vi "Public SV.vi"(0 "reference in":refnum<class "Stand.lvclass">, 11 "error in (no error)":errorcluster) -> (4 "reference out":refnum<class "Stand.lvclass">, 12 "dt public sv":u32, 15 "error out":errorcluster)   [LabVIEW 2019, in "Stand.lvclass"]
uses:
  Stand.lvclass
  C:/Users/ANENKOV_V1/Desktop/src/Device_class/Device.lvclass
  Stand.lvclass/Stand.ctl
  Device_class/Device.lvclass/Device.ctl
  DI_class/DI.lvclass/DI.ctl
  SV_Puplisher_class/SV_Publisher.lvclass/SV_Publisher.ctl
  FPGA/TypeDef/AI index.ctl
  AI_class/AI.lvclass/AI.ctl
  AnalogComparator_class/AnalogComparator.lvclass/AnalogComparator.ctl
  TypeDef/State Engine.ctl
  PM_Group_class/PM_Group.lvclass/PM_Group.ctl
  Engine_1DO_2DI_class/Engine_1DO_2DI.lvclass/Engine_1DO_2DI.ctl
  Valve_2DO_2DI_class/Valve_2DO_2DI.lvclass/Valve_2DO_2DI.ctl
  SV_Puplisher_class/Set SV.vi/1ae5d02c-efd0-450a-8aa4-8388e25d05bc.vi
  AnalogComparator_class/GetStatus.vi
  Engine_1DO_2DI_class/GetEngineState.vi
  Engine_1DO_2DI_class/Engine_1DO_2DI.lvclass
  OWEN HMI/Global - Data.vi
  FPGA_API_class/FPGA API.lvclass
  AI_class/AI.lvclass
  DI_class/DI.lvclass
  SV_Puplisher_class/SV_Publisher.lvclass
  Device_class/Device.lvclass
  PM_Group_class/PM_Group.lvclass
  ExpFitter/ExpFitter.lvclass
  OWEN HMI/OWEN HMI.lvclass
  Valve_2DO_2DI_class/Valve_2DO_2DI.lvclass
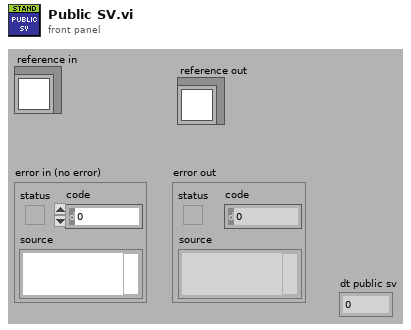
[diagram p1: front panel]
types:
  T1 = typedef "AI index.ctl" = u8
  T2 = typedef "AI_Data.ctl" = cluster{"Stat Data":T3, "OutOfRangeMax":bool, "OutOfRangeMin":bool, "HIHI":bool, "HI":bool, "LO":bool, "LOLO":bool}
  T3 = typedef "AI Statistics Data.ctl" = cluster{"raw mean":dbl, "scl mean":dbl, "raw mean 1Hz":dbl, "scl mean 1Hz":dbl}
  T4 = typedef "State Engine.ctl" = enum16{"Unknown", "Off", "TupningOn", "On", "TurningOff"}
  T5 = typedef "State PMG.ctl" = cluster{"PMG Mode":T6, "M12":T7, "M21":T7, "M24":T7}
  T6 = typedef "PMG Mode.ctl" = enum16{"Idel", "Filling", "Pressure"}
  T7 = typedef "State Engine 2.ctl" = cluster{"EngState":T4, "Active":bool, "Contactor":bool, "CMD":bool, "Automat":bool}
  T8 = typedef "Data Stand.ctl" = cluster{"CommCounter":u64, "BeginFilingLevel":dbl, "SP DUT":dbl, "SP CHAMBER":dbl, "Mode":T9, "ExecuteStepState":T10, "Direction":T11, "Direction Filling":T11, "STS":T12, "SP_TYPE_DUT":T13, "SP_TYPE_CHAMBER":T13, "New Step":bool, "BURETE_TIME":u16, "With BURETE":bool, "With Nitro":bool, "State 44-1-2":T14, "Measure leak":bool, "hold":bool}
  T9 = typedef "Mode.ctl" = enum16{"IDLE", "FILLING", "EXECUTE_SP", "DRAIN"}
  T10 = typedef "ExecuteStepState.ctl" = enum16{"Init", "Set: Backpressure ", "Preload: HI", "Set: HI", "Maintenance: HI", "Down: Pressure", "BLOCK"}
  T11 = typedef "Direction.ctl" = enum8{"DUT", "Chamber"}
  T12 = typedef "STS REG.ctl" = cluster{"IDLE":bool, "RYADY":bool, "STEP":bool, "ALARM":bool, "WARNING":bool, "REMOTE":bool, "SP_EXEC_DONE_DUT":bool, "SP_EXEC_DONE_CHAMBER":bool, "FILING_DONE_DUT":bool, "FILING_DONE_CHAMBER":bool, "BURETE_STATE":bool}
  T13 = typedef "SP_TYPE.ctl" = enum16{"ERROR", "ZIRO", "BASE", "SP"}
  T14 = typedef "State 44-1-2.ctl" = enum16{"Init", "Idle", "Wait", "Open 44-1", "Open 44-2", "Close 44-1", "Close 44-2"}
  T15 = typedef "DataExpFit.ctl" = cluster{"amplitude":dbl, "damping":dbl, "offset":dbl, "residue":dbl, "valid":bool, "T [s]":dbl}
  T16 = typedef "valveState.ctl" = enum16{"Unknown", "Closed", "Opening", "Opened", "Closing"}
  T17 = typedef "Setting Stand.ctl" = cluster{"Pressure Source":T18, "dt pressure down ms":i32, "dP pressure down MPa":dbl, "Haskel":T19, "Pump":T19, "Accuracy [%]":dbl, "Accuracy max [MPa]":dbl, "Accuracy min [MPa]":dbl, "BackPressurVoltage [V]":dbl}
  T18 = typedef "Pressure Source.ctl" = enum16{"Internal", "Modbus", "UDP"}
  T19 = typedef "Setting Pressure PI.ctl" = cluster{"A [MPa/V]":dbl, "P0 [MPa]":dbl}
  T20 = typedef "TCP Slave.lvclass/Connection.ctl" = cluster{"Connected?":bool, "IP address":string, "connection error":errorcluster}
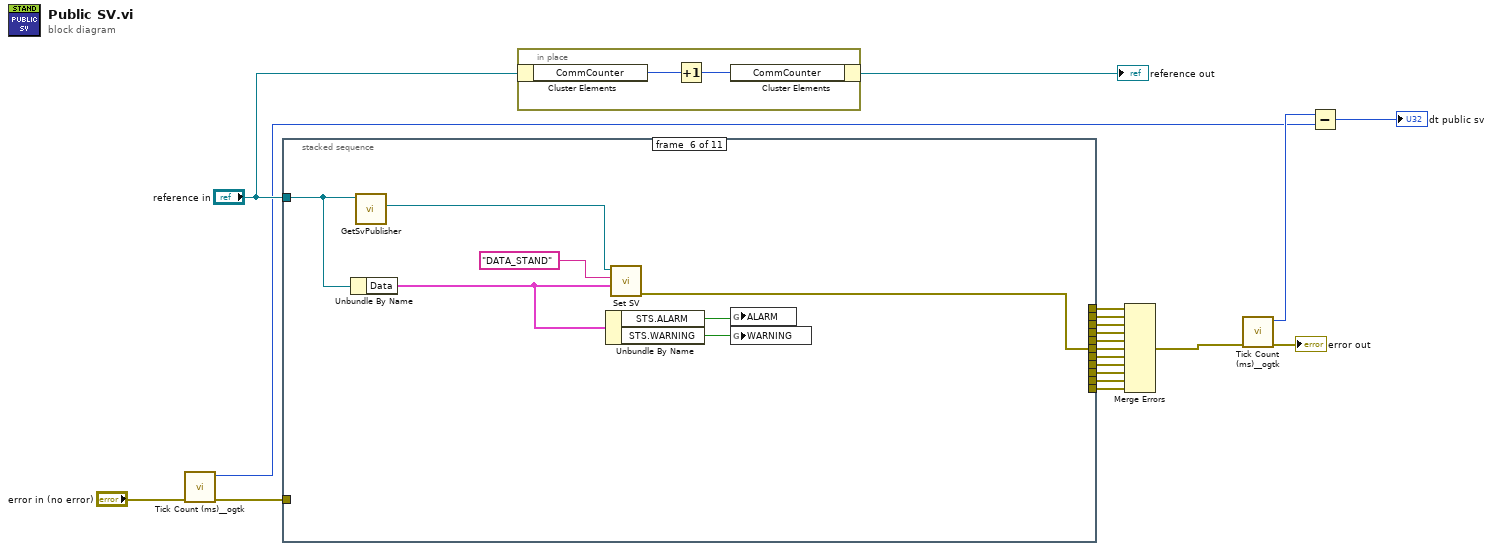
[diagram p0: block diagram]
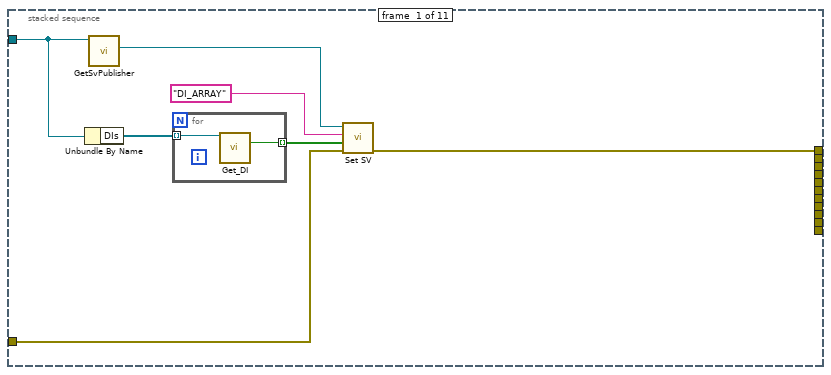
[diagram p2: hidden frame]
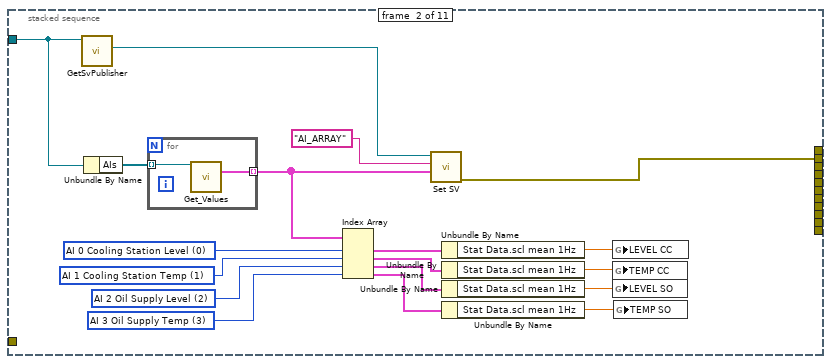
[diagram p3: hidden frame]
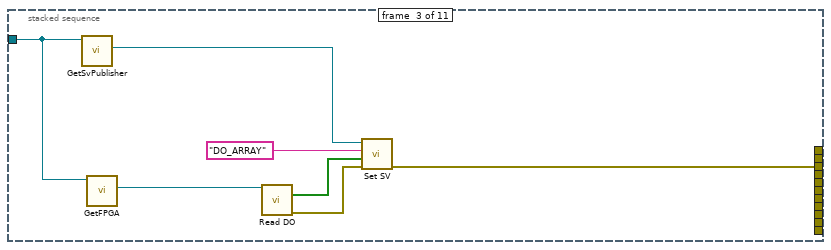
[diagram p4: hidden frame]
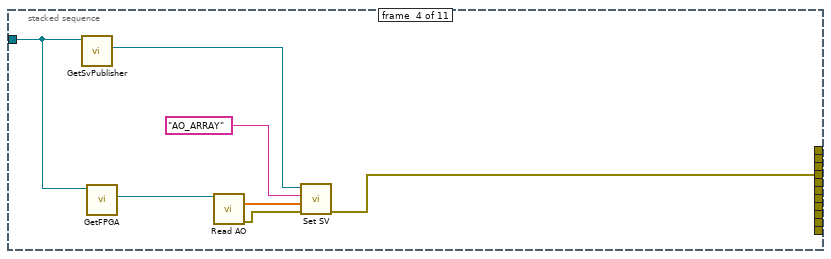
[diagram p5: hidden frame]
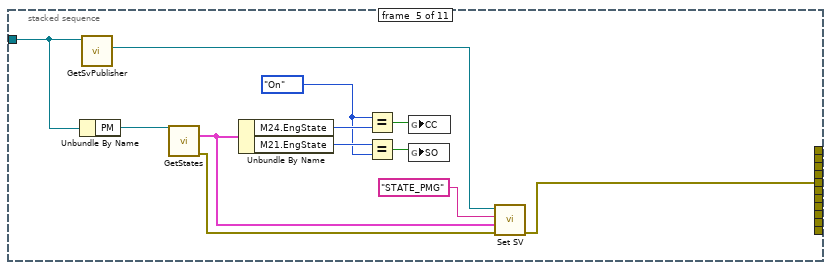
[diagram p6: hidden frame]
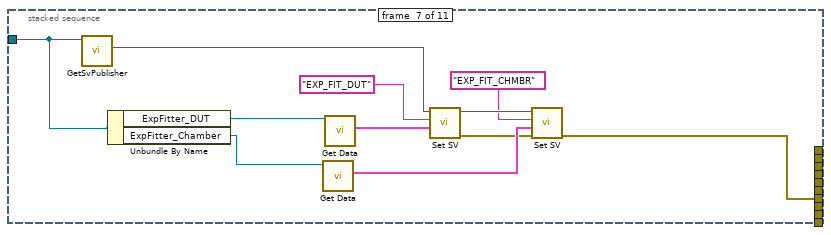
[diagram p7: hidden frame]
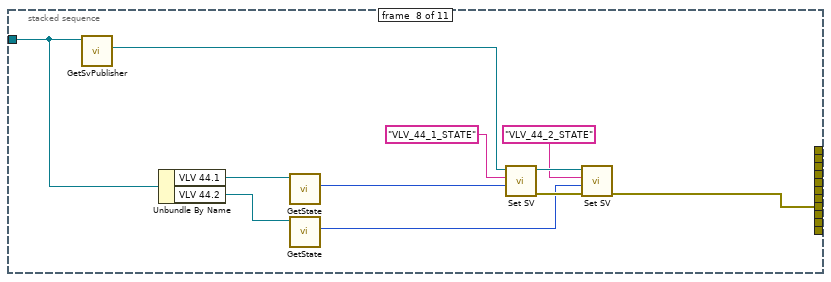
[diagram p8: hidden frame]
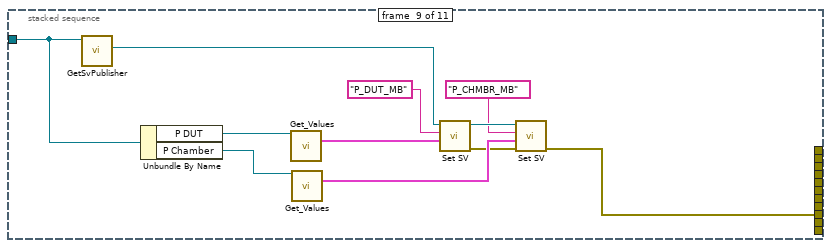
[diagram p9: hidden frame]
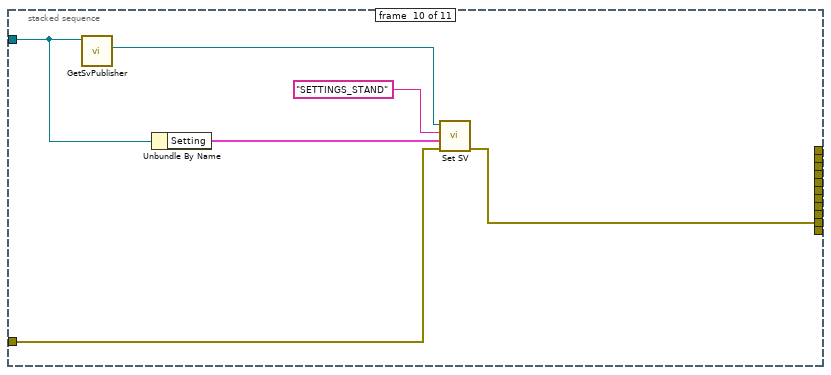
[diagram p10: hidden frame]
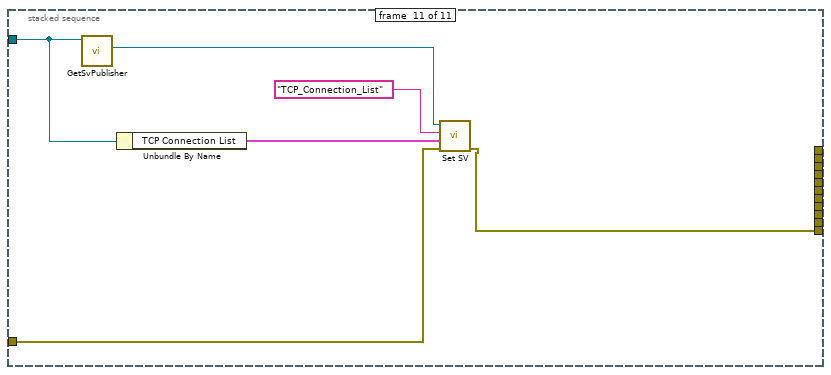
[diagram p11: hidden frame]
diagram:
  n1 = call <userlib>:"Tick Count (ms)__ogtk.vi"("error in (no error)"="error in (no error)") -> ("error out"=w13:errorcluster, "millisecond timer value"=w14:u32)  [unwired: 9 in]
  n2 = stacked-sequence {
    tunnel: "reference in" -> [w25 w47 w54 w63 w75 w82 w93 w96 w107 w120 w126]
    tunnel: w13 -> [w21 _ _ _ _ _ _ _ _ w116 w123]
    tunnel: [w22 _ _ _ _ _ _ _ _ _ _] -> w12
    tunnel: [_ w30 _ _ _ _ _ _ _ _ _] -> w10
    tunnel: [_ _ w50 _ _ _ _ _ _ _ _] -> w9
    tunnel: [_ _ _ w57 _ _ _ _ _ _ _] -> w8
    tunnel: [_ _ _ _ w64 _ _ _ _ _ _] -> w7
    tunnel: [_ _ _ _ _ w79 _ _ _ _ _] -> w6
    tunnel: [_ _ _ _ _ _ w83 _ _ _ _] -> w5
    tunnel: [_ _ _ _ _ _ _ w94 _ _ _] -> w4
    tunnel: [_ _ _ _ _ _ _ _ w105 _ _] -> w3
    tunnel: [_ _ _ _ _ _ _ _ _ w117 _] -> w2
    tunnel: [_ _ _ _ _ _ _ _ _ _ w122] -> w1
    frame #0 {
      n3 = Unbundle By Name(w25) -> ("DIs"=w24:refnum<class "DI.lvclass">[])
      n4 = call "GetSvPublisher.vi"("Device in"=w25) -> ("SV_Publisher.lvclass"=w23:refnum<class "SV_Publisher.lvclass">)  [unwired: 10 in]
      n5 = for {
        tunnel: w24 -> [w29] mode=indexing
        tunnel: [w28] -> w27 mode=indexing
        n6 = call "Get_DI.vi"("reference in"=w29) -> ("DI"=w28:bool)  [unwired: 14 in]
      }
      n7 = call "Set SV.vi"("error in (no error)"=w21, "SV Value"=w27, "SV Name"="DI_ARRAY", "SV_Publisher in"=w23) -> ("error out"=w22:errorcluster)  [unwired: 6 in, 1 out]
    }
    frame #1 {
      w34 = T1 3 items=["AI 0 Cooling Station Level", "AI 1 Cooling Station Temp", "AI 2 Oil Supply Level", "AI 3 Oil Supply Temp", "AI 4 ", "AI 5 Pressure Haskel", "AI 6 Pressure DUT", "AI 7 Pressure Chamber", "AI 8 Pressure Air inlet", "AI 9 Pressure Air outlet", "AI 10 Pressure Messure Line"] ("AI index")
      w35 = T1 2 items=["AI 0 Cooling Station Level", "AI 1 Cooling Station Temp", "AI 2 Oil Supply Level", "AI 3 Oil Supply Temp", "AI 4 ", "AI 5 Pressure Haskel", "AI 6 Pressure DUT", "AI 7 Pressure Chamber", "AI 8 Pressure Air inlet", "AI 9 Pressure Air outlet", "AI 10 Pressure Messure Line"] ("AI index")
      w36 = T1 1 items=["AI 0 Cooling Station Level", "AI 1 Cooling Station Temp", "AI 2 Oil Supply Level", "AI 3 Oil Supply Temp", "AI 4 ", "AI 5 Pressure Haskel", "AI 6 Pressure DUT", "AI 7 Pressure Chamber", "AI 8 Pressure Air inlet", "AI 9 Pressure Air outlet", "AI 10 Pressure Messure Line"] ("AI index")
      w37 = T1 0 items=["AI 0 Cooling Station Level", "AI 1 Cooling Station Temp", "AI 2 Oil Supply Level", "AI 3 Oil Supply Temp", "AI 4 ", "AI 5 Pressure Haskel", "AI 6 Pressure DUT", "AI 7 Pressure Chamber", "AI 8 Pressure Air inlet", "AI 9 Pressure Air outlet", "AI 10 Pressure Messure Line"] ("AI index")
      n8 = call "GetSvPublisher.vi"("Device in"=w47) -> ("SV_Publisher.lvclass"=w31:refnum<class "SV_Publisher.lvclass">)  [unwired: 10 in]
      n9 = Unbundle By Name(w47) -> ("AIs"=w32:refnum<class "AI.lvclass">[])
      n10 = for {
        tunnel: w32 -> [w49] mode=indexing
        tunnel: [w48] -> w38 mode=indexing
        n11 = call "Get_Values.vi"("reference in"=w49) -> ("Data"=w48:T2)  [unwired: 14 in]
      }
      n12 = Index Array(array=w38, index #1=w37, index #2=w36, index #3=w35, index #4=w34) -> (element #1=w39:T2, element #2=w40:T2, element #3=w41:T2, element #4=w42:T2)
      n13 = call "Set SV.vi"("SV Value"=w38, "SV Name"="AI_ARRAY", "SV_Publisher in"=w31) -> ("error out"=w30:errorcluster)  [unwired: 7 in, 1 out]
      n14 = Unbundle By Name(w39) -> ("Stat Data.scl mean 1Hz"=w43:dbl)
      n15 = Unbundle By Name(w40) -> ("Stat Data.scl mean 1Hz"=w46:dbl)
      n16 = Unbundle By Name(w41) -> ("Stat Data.scl mean 1Hz"=w45:dbl)
      n17 = Unbundle By Name(w42) -> ("Stat Data.scl mean 1Hz"=w44:dbl)
      n18 = global write "Global - Data.vi" "LEVEL CC"(w43) -> ()
      n19 = global write "Global - Data.vi" "TEMP CC"(w46) -> ()
      n20 = global write "Global - Data.vi" "LEVEL SO"(w45) -> ()
      n21 = global write "Global - Data.vi" "TEMP SO"(w44) -> ()
    }
    frame #2 {
      n22 = call "GetSvPublisher.vi"("Device in"=w54) -> ("SV_Publisher.lvclass"=w52:refnum<class "SV_Publisher.lvclass">)  [unwired: 10 in]
      n23 = call "GetFPGA.vi"("Device in"=w54) -> ("FPGA API.lvclass"=w53:refnum<class "FPGA API.lvclass">)  [unwired: 10 in]
      n24 = call-dynamic "Read DO.vi"("FPGA API in"=w53) -> ("Ds"=w56:bool[], "error out"=w51:errorcluster)  [unwired: 12 in, 1 out]
      n25 = call "Set SV.vi"("error in (no error)"=w51, "SV Value"=w56, "SV Name"="DO_ARRAY", "SV_Publisher in"=w52) -> ("error out"=w50:errorcluster)  [unwired: 6 in, 1 out]
    }
    frame #3 {
      n26 = call "GetSvPublisher.vi"("Device in"=w63) -> ("SV_Publisher.lvclass"=w59:refnum<class "SV_Publisher.lvclass">)  [unwired: 10 in]
      n27 = call "GetFPGA.vi"("Device in"=w63) -> ("FPGA API.lvclass"=w60:refnum<class "FPGA API.lvclass">)  [unwired: 10 in]
      n28 = call-dynamic "Read AO.vi"("FPGA API in"=w60) -> ("AO"=w62:dbl[], "error out"=w58:errorcluster)  [unwired: 12 in, 1 out]
      n29 = call "Set SV.vi"("error in (no error)"=w58, "SV Value"=w62, "SV Name"="AO_ARRAY", "SV_Publisher in"=w59) -> ("error out"=w57:errorcluster)  [unwired: 6 in, 1 out]
    }
    frame #4 {
      w69 = State_Engine."On" ("x")
      n30 = Unbundle By Name(w75) -> ("PM"=w67:refnum<class "PM_Group.lvclass">)
      n31 = call "GetSvPublisher.vi"("Device in"=w75) -> ("SV_Publisher.lvclass"=w65:refnum<class "SV_Publisher.lvclass">)  [unwired: 10 in]
      n32 = call "GetStates.vi"("Pump_1AI_1DO_2DI in"=w67) -> ("PMG"=w74:T5, "error out"=w66:errorcluster)  [unwired: 13 in]
      n33 = Unbundle By Name(w74) -> ("M24.EngState"=w70:T4, "M21.EngState"=w72:T4)
      n34 = Equal?(x=w69, y=w70) -> (x = y?=w71:bool)
      n35 = Equal?(x=w72, y=w69) -> (x = y?=w73:bool)
      n36 = global write "Global - Data.vi" "CC"(w71) -> ()
      n37 = global write "Global - Data.vi" "SO"(w73) -> ()
      n38 = call "Set SV.vi"("error in (no error)"=w66, "SV Value"=w74, "SV Name"="STATE_PMG", "SV_Publisher in"=w65) -> ("error out"=w64:errorcluster)  [unwired: 6 in, 1 out]
    }
    frame #5 {
      n39 = Unbundle By Name(w82) -> ("Data"=w78:T8)
      n40 = call "GetSvPublisher.vi"("Device in"=w82) -> ("SV_Publisher.lvclass"=w80:refnum<class "SV_Publisher.lvclass">)  [unwired: 10 in]
      n41 = Unbundle By Name(w78) -> ("STS.ALARM"=w77:bool, "STS.WARNING"=w76:bool)
      n42 = call "Set SV.vi"("SV Value"=w78, "SV Name"="DATA_STAND", "SV_Publisher in"=w80) -> ("error out"=w79:errorcluster)  [unwired: 7 in, 1 out]
      n43 = global write "Global - Data.vi" "ALARM"(w77) -> ()
      n44 = global write "Global - Data.vi" "WARNING"(w76) -> ()
    }
    frame #6 {
      n45 = call "GetSvPublisher.vi"("Device in"=w93) -> ("SV_Publisher.lvclass"=w84:refnum<class "SV_Publisher.lvclass">)  [unwired: 10 in]
      n46 = Unbundle By Name(w93) -> ("ExpFitter_DUT"=w86:refnum<class "ExpFitter.lvclass">, "ExpFitter_Chamber"=w85:refnum<class "ExpFitter.lvclass">)
      n47 = call "Get Data.vi"("ExpFitter in"=w85) -> ("DataExpFit"=w92:T15)  [unwired: 10 in]
      n48 = call "Get Data.vi"("ExpFitter in"=w86) -> ("DataExpFit"=w91:T15)  [unwired: 10 in]
      n49 = call "Set SV.vi"("SV Value"=w91, "SV Name"="EXP_FIT_DUT", "SV_Publisher in"=w84) -> ("error out"=w89:errorcluster, "SV_Publisher out"=w90:refnum<class "SV_Publisher.lvclass">)  [unwired: 7 in]
      n50 = call "Set SV.vi"("error in (no error)"=w89, "SV Value"=w92, "SV Name"="EXP_FIT_CHMBR", "SV_Publisher in"=w90) -> ("error out"=w83:errorcluster)  [unwired: 6 in, 1 out]
    }
    frame #7 {
      n51 = call "GetSvPublisher.vi"("Device in"=w96) -> ("SV_Publisher.lvclass"=w95:refnum<class "SV_Publisher.lvclass">)  [unwired: 10 in]
      n52 = Unbundle By Name(w96) -> ("VLV 44.1"=w104:refnum<class "Valve_2DO_2DI.lvclass">, "VLV 44.2"=w103:refnum<class "Valve_2DO_2DI.lvclass">)
      n53 = call "GetState.vi"("Pump_1AI_1DO_2DI in"=w104) -> ("valveState"=w99:T16)  [unwired: 10 in]
      n54 = call "GetState.vi"("Pump_1AI_1DO_2DI in"=w103) -> ("valveState"=w100:T16)  [unwired: 10 in]
      n55 = call "Set SV.vi"("SV Value"=w99, "SV Name"="VLV_44_1_STATE", "SV_Publisher in"=w95) -> ("error out"=w101:errorcluster, "SV_Publisher out"=w102:refnum<class "SV_Publisher.lvclass">)  [unwired: 7 in]
      n56 = call "Set SV.vi"("error in (no error)"=w101, "SV Value"=w100, "SV Name"="VLV_44_2_STATE", "SV_Publisher in"=w102) -> ("error out"=w94:errorcluster)  [unwired: 6 in, 1 out]
    }
    frame #8 {
      n57 = call "GetSvPublisher.vi"("Device in"=w107) -> ("SV_Publisher.lvclass"=w106:refnum<class "SV_Publisher.lvclass">)  [unwired: 10 in]
      n58 = Unbundle By Name(w107) -> ("P DUT"=w110:refnum<class "AI.lvclass">, "P Chamber"=w111:refnum<class "AI.lvclass">)
      n59 = call "Get_Values.vi"("reference in"=w110) -> ("Data"=w115:T2)  [unwired: 14 in]
      n60 = call "Get_Values.vi"("reference in"=w111) -> ("Data"=w114:T2)  [unwired: 14 in]
      n61 = call "Set SV.vi"("SV Value"=w115, "SV Name"="P_DUT_MB", "SV_Publisher in"=w106) -> ("error out"=w112:errorcluster, "SV_Publisher out"=w113:refnum<class "SV_Publisher.lvclass">)  [unwired: 7 in]
      n62 = call "Set SV.vi"("error in (no error)"=w112, "SV Value"=w114, "SV Name"="P_CHMBR_MB", "SV_Publisher in"=w113) -> ("error out"=w105:errorcluster)  [unwired: 6 in, 1 out]
    }
    frame #9 {
      n63 = call "GetSvPublisher.vi"("Device in"=w120) -> ("SV_Publisher.lvclass"=w119:refnum<class "SV_Publisher.lvclass">)  [unwired: 10 in]
      n64 = Unbundle By Name(w120) -> ("Setting"=w118:T17)
      n65 = call "Set SV.vi"("error in (no error)"=w116, "SV Value"=w118, "SV Name"="SETTINGS_STAND", "SV_Publisher in"=w119) -> ("error out"=w117:errorcluster)  [unwired: 6 in, 1 out]
    }
    frame #10 {
      n66 = call "GetSvPublisher.vi"("Device in"=w126) -> ("SV_Publisher.lvclass"=w125:refnum<class "SV_Publisher.lvclass">)  [unwired: 10 in]
      n67 = Unbundle By Name(w126) -> ("TCP Connection List"=w124:T20[])
      n68 = call "Set SV.vi"("error in (no error)"=w123, "SV Value"=w124, "SV Name"="TCP_Connection_List", "SV_Publisher in"=w125) -> ("error out"=w122:errorcluster)  [unwired: 6 in, 1 out]
    }
  }
  n69 = in-place {
    n70 = in-place-cluster #1("reference in") -> ("CommCounter"=w129:u64)
    n71 = Increment(x=w129) -> (x+1=w128:u64)
    n72 = in-place-cluster #1("CommCounter"=w128) -> (→"reference out":refnum<class "Stand.lvclass">)
  }
  n73 = Merge Errors(w12, w10, w9, w8, w7, w6, w5, w4, w3, w2, w1) -> (w11:errorcluster)
  n74 = call <userlib>:"Tick Count (ms)__ogtk.vi"("error in (no error)"=w11) -> ("error out"=→"error out":errorcluster, "millisecond timer value"=w17:u32)  [unwired: 9 in]
  n75 = Subtract(x=w17, y=w14) -> (x-y=→"dt public sv":u32)
